vi "file int.vi"(8 "error in (no error)":errorcluster, 9 "number_of_points":i32, 10 "path":string, 11 "field":T1) -> (0 "error out":errorcluster, 3 "field out":T1)   [LabVIEW 2012, in "LightPipes.lvlib"]
doc: "__declspec(dllexport) void file_int(FIELD* field, const char* path, int number_of_points);"
uses:
  LightPipes.lvlib
  Debug/LightPipes.dll
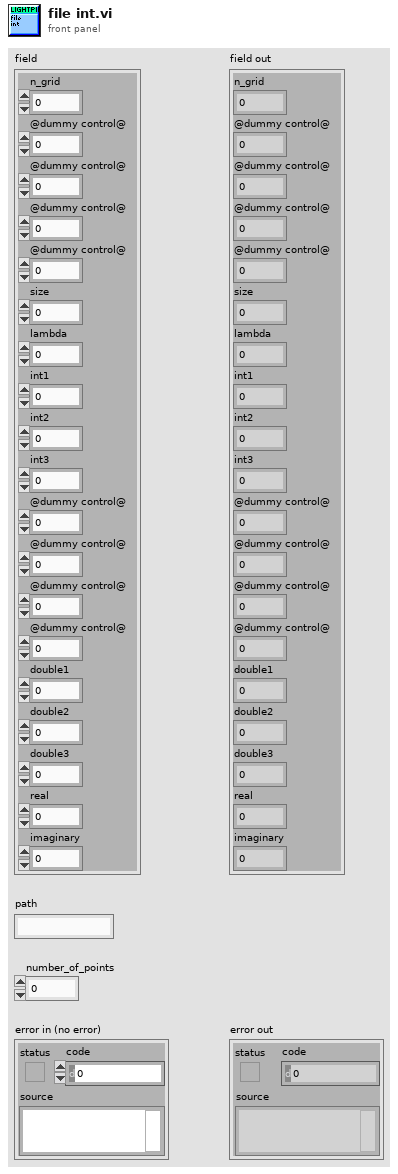
[diagram p1: front panel]
types:
  T1 = cluster{"n_grid":i32, "@dummy control@":i8, "@dummy control@":i8, "@dummy control@":i8, "@dummy control@":i8, "size":dbl, "lambda":dbl, "int1":i32, "int2":i32, "int3":i32, "@dummy control@":i8, "@dummy control@":i8, "@dummy control@":i8, "@dummy control@":i8, "double1":dbl, "double2":dbl, "double3":dbl, "real":u32, "imaginary":u32}
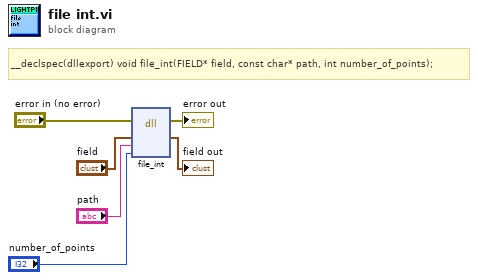
[diagram p0: block diagram]
diagram:
  # "__declspec(dllexport) void file_int(FIELD* field, const char* path, int number_of_points);"
  n1 = dll-call lib="C:/Users/Green Beret/Documents/Visual Studio 2012/Projects/LightPipes/Debug/LightPipes.*" fn="file_int"(error in="error in (no error)", "field"="field", "path"="path", "number_of_points"="number_of_points") -> (error out=→"error out":errorcluster, "field"=→"field out":T1)  [unwired: 5 in, 1 out]
